vi "Channels.vi"(5 "Ground level BP-filter width, Hz":dbl=5.0 format="%#_13g", 6 "Generator frequency, Hz":dbl format="%#_13g", 7 "Noise filter ratio":dbl=0.9 format="%#_13g", 8 "Noise high cutoff, Hz":dbl=10000.0 format="%#_13g", 9 "Sampling rate, Hz":dbl=100000.0 format="%#_13g", 10 "Number of samplings":i32) -> (0 "Field":dbl[](array[numeric]), 1 "Background":dbl[](array[numeric]), 2 "Differential":dbl[](array[numeric]), 3 "Time":dbl[](array[numeric]), 4 "Noise low cutoff":dbl=9950.0 format="%#_13g")   [LabVIEW 2015]
uses:
  <vilib>/Analysis/3filter.llb/Butterworth Filter (DBL).vi
  <vilib>/Analysis/NI_AALBase.lvlib
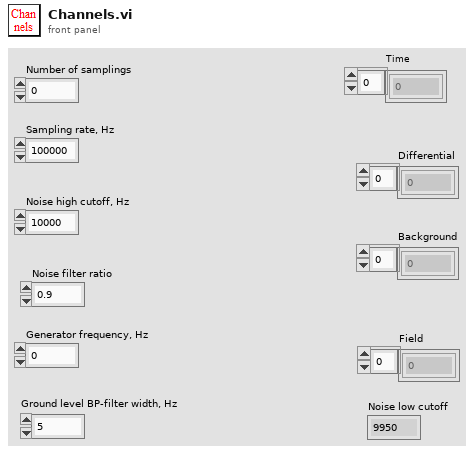
[diagram p1: front panel]
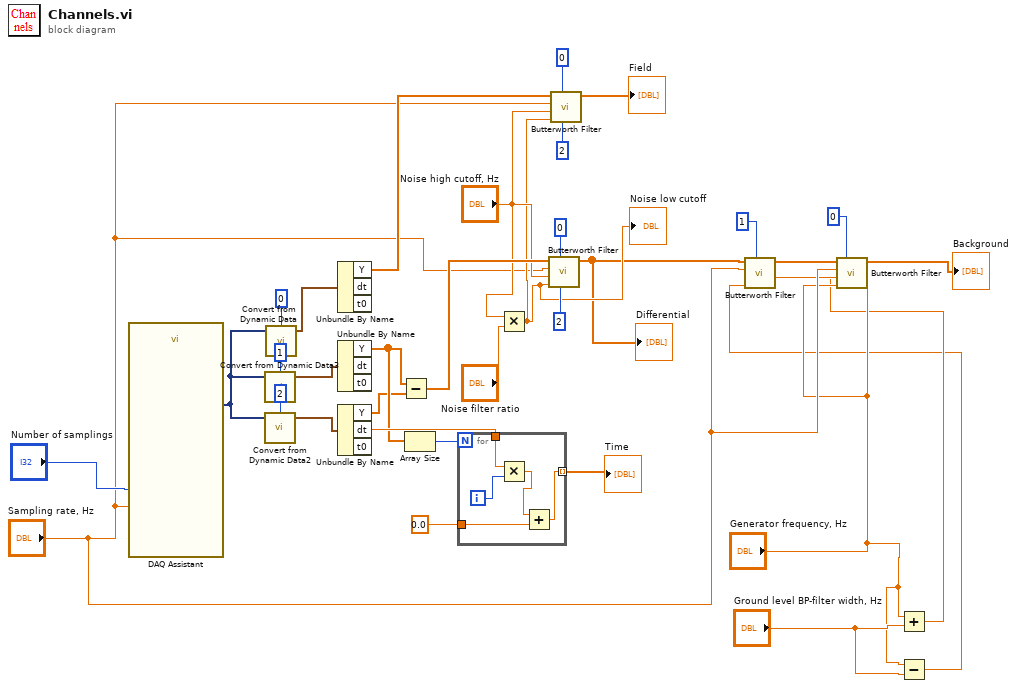
[diagram p0: block diagram]
diagram:
  n1 = call "DAQ Assistant"("rate"="Sampling rate, Hz", "number of samples"="Number of samplings") -> ("data"=w31:dynamicdata)  [unwired: 15 in, 2 out]
  n2 = call "Convert from Dynamic Data3"("Dynamic Data Type"=w31, "Channel"=1) -> ("Waveform"=w29:waveform(dbl))  [unwired: 2 in]
  n3 = call "Convert from Dynamic Data2"("Dynamic Data Type"=w31, "Channel"=2) -> ("Waveform"=w28:waveform(dbl))  [unwired: 2 in]
  n4 = call "Convert from Dynamic Data"("Dynamic Data Type"=w31, "Channel"=0) -> ("Waveform"=w30:waveform(dbl))  [unwired: 2 in]
  n5 = Unbundle By Name(w30) -> ("Y"=w16:dbl[])  [unwired: 2 out]
  n6 = Unbundle By Name(w29) -> ("Y"=w24:dbl[])  [unwired: 2 out]
  n7 = Unbundle By Name(w28) -> ("Y"=w23:dbl[], "dt"=w26:dbl)  [unwired: 1 out]
  n8 = Subtract(x=w24, y=w23) -> (x-y=w21:dbl[])
  n9 = Array Size(array=w24) -> (size(s)=w25:i32)
  n10 = for {
    N: w25 -> [_]
    tunnel: w26 -> [w38]
    tunnel: [w37] -> w11 mode=indexing
    tunnel: 0.0 -> [w35]
    i -> [w39]
    n11 = Multiply(x=w38, y=w39) -> (x*y=w36:dbl)
    n12 = Add(x=w36, y=w35) -> (x+y=w37:dbl)
  }
  "Time" <- w11
  n13 = Multiply(x="Noise high cutoff, Hz", y="Noise filter ratio") -> (x*y=w14:dbl)
  "Noise low cutoff" <- w14
  n14 = call-poly <vilib>:"Butterworth Filter.vi"("order"=2, "filter type"=0, "low cutoff freq: fl"=w14, "high cutoff freq: fh"="Noise high cutoff, Hz", "sampling freq: fs"="Sampling rate, Hz", "X"=w21) -> ("Filtered X"=w10:dbl[])  [unwired: 2 in, 1 out]
  "Differential" <- w10
  n15 = call-poly <vilib>:"Butterworth Filter.vi"("order"=2, "filter type"=0, "low cutoff freq: fl"=w14, "high cutoff freq: fh"="Noise high cutoff, Hz", "sampling freq: fs"="Sampling rate, Hz", "X"=w16) -> ("Filtered X"=→"Field":dbl[])  [unwired: 2 in, 1 out]
  n16 = Add(x="Generator frequency, Hz", y="Ground level BP-filter width, Hz") -> (x+y=w2:dbl)
  n17 = Subtract(x="Generator frequency, Hz", y="Ground level BP-filter width, Hz") -> (x-y=w1:dbl)
  n18 = call-poly <vilib>:"Butterworth Filter.vi"("filter type"=1, "low cutoff freq: fl"=w1, "high cutoff freq: fh"="Generator frequency, Hz", "sampling freq: fs"="Sampling rate, Hz", "X"=w10) -> ("Filtered X"=w9:dbl[])  [unwired: 3 in, 1 out]
  n19 = call-poly <vilib>:"Butterworth Filter.vi"("filter type"=0, "low cutoff freq: fl"="Generator frequency, Hz", "high cutoff freq: fh"=w2, "sampling freq: fs"="Sampling rate, Hz", "X"=w9) -> ("Filtered X"=→"Background":dbl[])  [unwired: 3 in, 1 out]
